vi "Move stage.vi"(4 "error in":errorcluster, 5 "input main cluster":T2, 7 "Cursor.Cursor Position":T1) -> (0 "error out":errorcluster, 1 "output main cluster":T2)   [LabVIEW 2010]
uses:
  Main_cluster.ctl
  <vilib>/vision/Image Controls.llb/IMAQ Image.ctl
  <vilib>/Utility/miscctls.llb/LVPointDoubleTypeDef.ctl
  <vilib>/DAQmx/write.llb/DAQmx Write (Analog DBL 1Chan 1Samp).vi
  <vilib>/daqmx/miscellaneous.llb/DAQmx Fill In Error Info.vi
  PI E710 Stage.lvlib
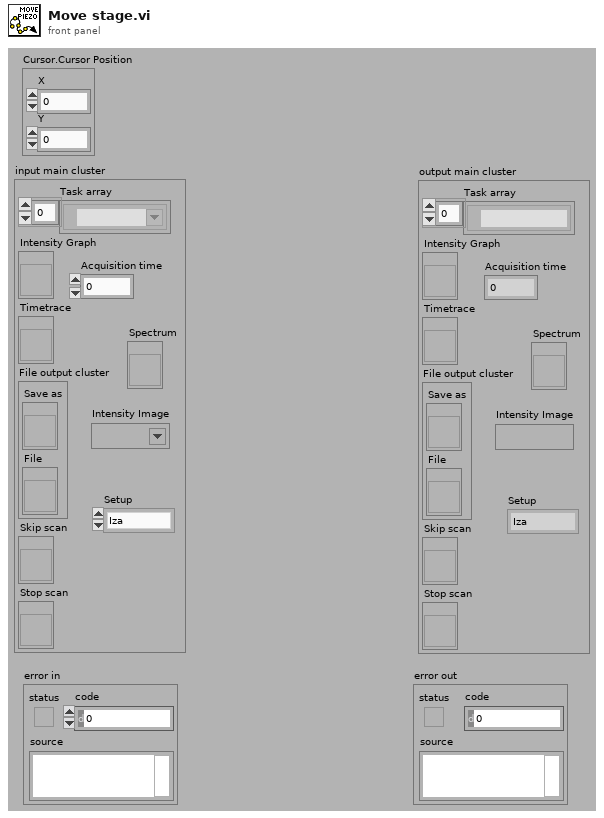
[diagram p1: front panel]
types:
  T1 = typedef "LVPointDoubleTypeDef.ctl" = cluster{"X":dbl, "Y":dbl}
  T2 = typedef "Main_cluster.ctl" = cluster{"Task array":refnum<k21>[], "Intensity Graph":refnum<vi>, "Timetrace":refnum<vi>, "File output cluster":cluster{"Save as":refnum<vi>, "File":refnum<vi>}, "Skip scan":refnum<vi>, "Stop scan":refnum<vi>, "Acquisition time":dbl, "Setup":enum16{"Iza", "Lukasz"}, "Spectrum":refnum<vi>, "Intensity Image":T3}
  T3 = typedef "IMAQ Image.ctl" = refnum<image>
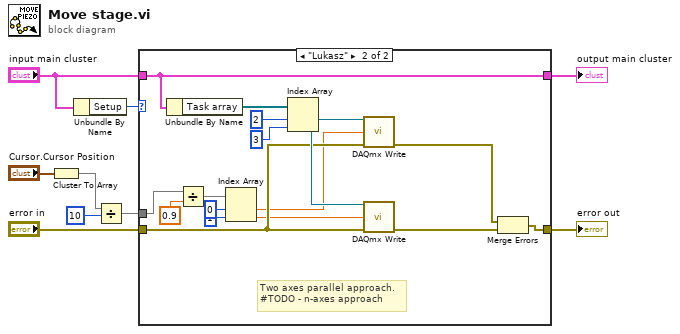
[diagram p0: block diagram]
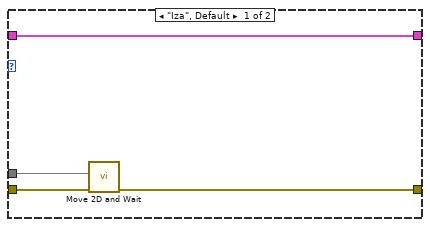
[diagram p2: hidden frame]
diagram:
  n1 = Cluster To Array(cluster="Cursor.Cursor Position") -> (array=w3:dbl[])
  n2 = Unbundle By Name("input main cluster") -> ("Setup"=w8:enum16{"Iza", "Lukasz"})
  n3 = Divide(x=w3, y=10 ("X")) -> (x/y=w2:dbl[])
  n4 = case shown="\"Lukasz\"" w8 {
    tunnel: [w10 w30] -> w7
    tunnel: "input main cluster" -> [w10 w30]
    tunnel: w2 -> [w13 w16]
    tunnel: "error in" -> [w12 w24]
    tunnel: [w11 w17] -> w4
    frame "Iza", Default {
      n5 = call "Move 2D and Wait.vi"("error IO"=w12, "Position table"=w13) -> ("error out"=w11:errorcluster)  [unwired: 5 in]
    }
    frame "Lukasz" {
      # "Two axes parallel approach.\n#TODO - n-axes approach"
      n6 = Unbundle By Name(w30) -> ("Task array"=w29:refnum<k21>[])
      n7 = Divide(x=w16, y=0.9) -> (x/y=w15:dbl[])
      n8 = Index Array(array=w15, index #1=0 ("index"), index #2=1 ("index")) -> (element #1=w21:dbl, element #2=w20:dbl)
      n9 = Index Array(array=w29, index #1=2 ("index"), index #2=3 ("index")) -> (element #1=w26:refnum<k21>, element #2=w25:refnum<k21>)
      n10 = call-poly <vilib>:"DAQmx Write.vi"("task/channels in"=w26, "data"=w21, "error in"=w24) -> ("error out"=w19:errorcluster)  [unwired: 10 in, 2 out]
      n11 = call-poly <vilib>:"DAQmx Write.vi"("task/channels in"=w25, "data"=w20, "error in"=w24) -> ("error out"=w18:errorcluster)  [unwired: 10 in, 2 out]
      n12 = Merge Errors(w19, w18) -> (w17:errorcluster)
    }
  }
  "output main cluster" <- w7
  "error out" <- w4
